vi "Log Error.vi"(8 "error in (no error)":errorcluster, 10 "Error":errorcluster, 11 "Controller in":refnum<class "Controller.lvclass">) -> (0 "error out":errorcluster, 3 "Controller out":refnum<class "Controller.lvclass">)   [LabVIEW 2022 SP3, in "Controller.lvlib" / "Controller.lvclass"]
uses:
  Controller.lvclass
  Controller.lvclass/Controller.ctl
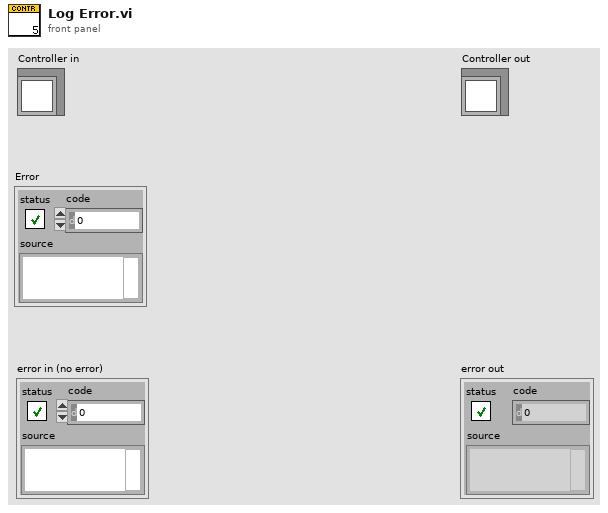
[diagram p1: front panel]
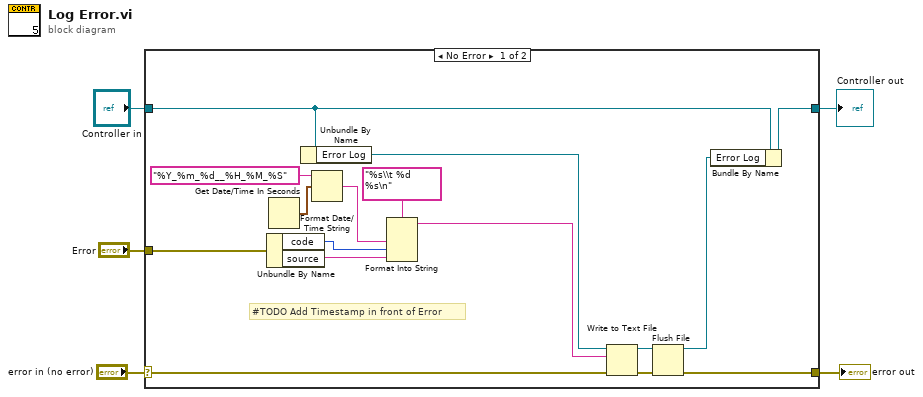
[diagram p0: block diagram]
diagram:
  n1 = case shown="No Error" "error in (no error)" {
    selector: "error in (no error)" -> [w21 w23]
    tunnel: [w13 w23] -> w4
    tunnel: [w17 w22] -> w2
    tunnel: "Controller in" -> [w19 w22]
    tunnel: "Error" -> [w16 _]
    frame No Error {
      # "#TODO Add Timestamp in front of Error"
      n2 = Unbundle By Name(w16) -> ("code"=w9:i32, "source"=w10:string)
      n3 = Get Date/Time In Seconds() -> (seconds since 1Jan1904=w7:timestamp)
      n4 = Unbundle By Name(w19) -> ("Error Log"=w18:refnum<file>)
      n5 = Format Date/Time String(time format string (%c)="%Y_%m_%d__%H_%M_%S", seconds (now)=w7) -> (date/time string=w6:string)  [unwired: 1 in]
      n6 = Format Into String(format string="%s\\t %d    %s\n", w6, w9, w10) -> (resulting string=w15:string)  [unwired: 2 in, 1 out]
      n7 = Write to Text File(file (use dialog)=w18, text=w15, error in=w21) -> (refnum out=w12:refnum<file>, error out=w20:errorcluster)  [unwired: 1 in, 1 out]
      n8 = Flush File(refnum=w12, error in=w20) -> (refnum out=w11:refnum<file>, error out=w13:errorcluster)
      n9 = Bundle By Name(cluster=w19, "Error Log"=w11) -> (w17:refnum<class "Controller.lvclass">)
    }
    frame Error {
    }
  }
  "error out" <- w4
  "Controller out" <- w2
